vi "MSEncoder Case-22-PhaseScanII.vi"(8 "error in (no error)":errorcluster, 9 "ParamValIn":variant, 11 "MSEncoder in":refnum<class "MSEncoder.lvclass">) -> (0 "error out":errorcluster, 3 "MSEncoder out":refnum<class "MSEncoder.lvclass">)   [LabVIEW 2018, in "MSEncoder.lvclass"]
uses:
  MSEncoder.lvclass
  Ctl/MSEditorParam phaseScanII.ctl
  PublicSubVI/Ctl/MathieuEqParam.ctl
  MSEncoder.lvclass/MSEncoder.ctl
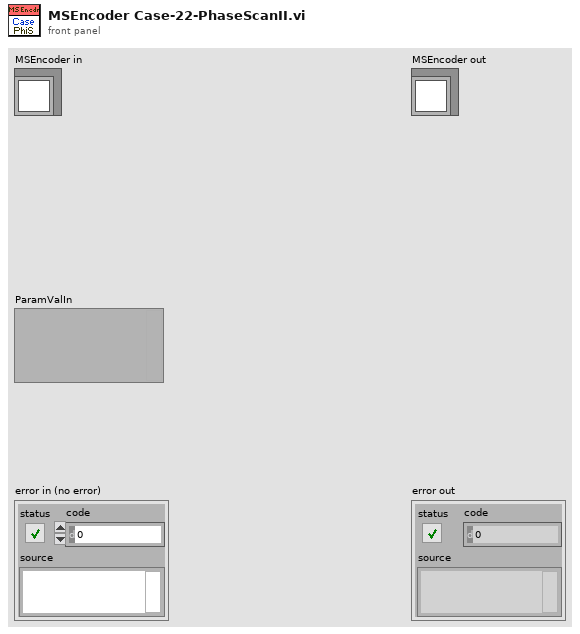
[diagram p1: front panel]
types:
  T1 = typedef "MSEditorParam phaseScanII.ctl" = cluster{"auxWfmType":u32, "auxStart":u32, "iauxCyc":ext, "auxCyc":ext, "beta":ext, "betaScale":ext, "auxAmp":ext, "auxPulse1":ext[], "auxPulse2":ext[], "auxPulseAmp":ext[], "dm":ext, "freq":ext[], "stepWidth":u32}
  T2 = cluster{"f1":ext, "m1":ext, "f2":ext, "Stepwise":u32, "dm":ext}
  T3 = typedef "MathieuEqParam.ctl" = cluster{"mz(Th)":ext, "Amp(V)":ext, "Freq(Hz)":ext, "Beta":ext, "r_0 (mm)":ext, "z_0 (mm)":ext}
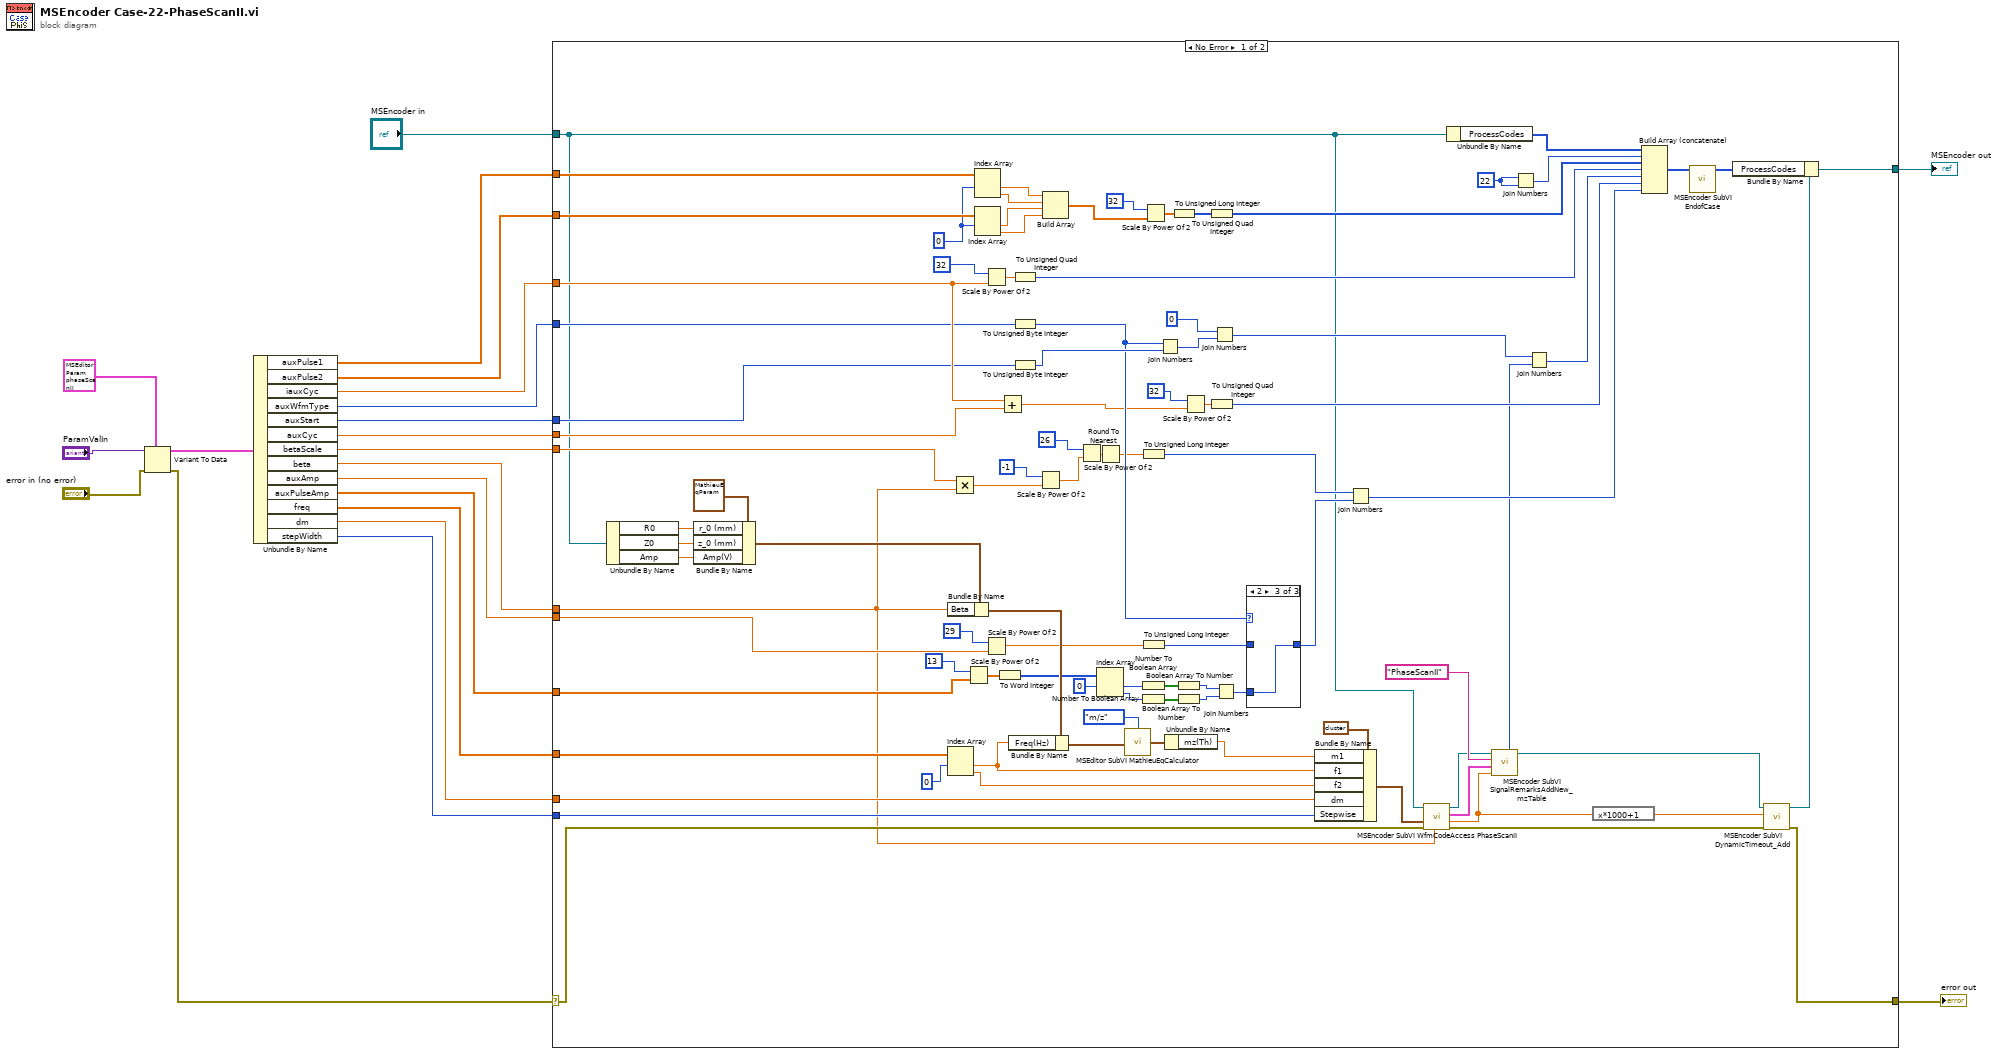
[diagram p0: block diagram]
diagram:
  n1 = Variant To Data(error in="error in (no error)", type=T1 {"auxWfmType"=0, "auxStart"=0, "iauxCyc"=0.0, "auxCyc"=0.0, "beta"=0.5, "betaScale"=1.0, "auxAmp"=1.0, "auxPulse1"=[0.0, 0.5], "auxPulse2"=[0.5, 1.0], "auxPulseAmp"=[1.0, -1.0], "dm"=1.0, "freq"=[100000.0, 50000.0], "stepWidth"=1} ("ParamValueType"), Variant="ParamValIn") -> (data=w3:T1, error out=w2:errorcluster)
  n2 = Unbundle By Name(w3) -> ("auxPulse1"=w20:ext[], "auxPulse2"=w19:ext[], "iauxCyc"=w18:ext, "auxWfmType"=w17:u32, "auxStart"=w16:u32, "auxCyc"=w15:ext, "betaScale"=w14:ext, "beta"=w13:ext, "auxAmp"=w12:ext, "auxPulseAmp"=w11:ext[], "freq"=w10:ext[], "dm"=w9:ext, "stepWidth"=w8:u32)
  n3 = case shown="No Error" w2 {
    selector: w2 -> [w37 w118]
    tunnel: "MSEncoder in" -> [w34 w117]
    tunnel: [w39 w118] -> w21
    tunnel: [w113 w117] -> w6
    tunnel: w20 -> [w107 _]
    tunnel: w19 -> [w106 _]
    tunnel: w18 -> [w105 _]
    tunnel: w17 -> [w104 _]
    tunnel: w16 -> [w103 _]
    tunnel: w15 -> [w102 _]
    tunnel: w14 -> [w101 _]
    tunnel: w13 -> [w22 _]
    tunnel: w12 -> [w100 _]
    tunnel: w11 -> [w99 _]
    tunnel: w10 -> [w98 _]
    tunnel: w9 -> [w26 _]
    tunnel: w8 -> [w25 _]
    frame No Error {
      w90 = u32 22
      w85 = 0 ("index")
      n4 = Unbundle By Name(w34) -> ("R0"=w112:ext, "Z0"=w111:ext, "Amp"=w110:ext)
      n5 = Bundle By Name(cluster=T3 {"mz(Th)"=0.0, "Amp(V)"=330.0, "Freq(Hz)"=0.0, "Beta"=1.0, "r_0 (mm)"=10.0, "z_0 (mm)"=7.0710678118654755} ("Parametres in"), "r_0 (mm)"=w112, "z_0 (mm)"=w111, "Amp(V)"=w110) -> (w108:T3)
      n6 = Bundle By Name(cluster=w108, "Beta"=w22) -> (w97:T3)
      n7 = Index Array(array=w98, index #1=0 ("index")) -> (element #1=w28:ext, element #2=w27:ext)  [unwired: 1 in]
      n8 = Multiply(x=w101, y=w22) -> (x*y=w57:ext)
      n9 = Scale By Power Of 2(n=i16 13, x=w99) -> (x*2^n=w55:ext[])
      n10 = Index Array(array=w107, index #1=w85) -> (element #1=w83:ext, element #2=w82:ext)  [unwired: 1 in]
      n11 = Index Array(array=w106, index #1=w85) -> (element #1=w81:ext, element #2=w80:ext)  [unwired: 1 in]
      n12 = Scale By Power Of 2(n=i16 32, x=w105) -> (x*2^n=w87:ext)
      n13 = Scale By Power Of 2(n=i16 29, x=w100) -> (x*2^n=w60:ext)
      n14 = To Word Integer(number=w55) -> (16bit integer=w54:i16[])
      n15 = Add(x=w105, y=w102) -> (x+y=w43:ext)
      n16 = Bundle By Name(cluster=w97, "Freq(Hz)"=w28) -> (w84:T3)
      n17 = To Unsigned Quad Integer(1:w87) -> (0:w74:u64)
      n18 = To Unsigned Byte Integer(number=w104) -> (unsigned 8bit integer=w47:u8)
      n19 = To Unsigned Byte Integer(number=w103) -> (unsigned 8bit integer=w73:u8)
      n20 = Scale By Power Of 2(n=i16 -1, x=w57) -> (x*2^n=w63:ext)
      n21 = Build Array(w83, w82, w81, w80) -> (w78:ext[])
      n22 = Scale By Power Of 2(n=i16 26, x=w63) -> (x*2^n=w61:ext)
      n23 = Round To Nearest(number=w61) -> (nearest integer value=w42:ext)
      n24 = Index Array(array=w54, index #1=0 ("index")) -> (element #1=w53:i16, element #2=w52:i16)  [unwired: 1 in]
      n25 = call "MSEditor SubVI MathieuEqCalculator.vi"("Target (Freq)"=enum16{"m/z", "Volt", "Freq", "Beta"}."m/z", "Parametres in"=w84) -> ("Parametres out"=w92:T3)  [unwired: 2 in]
      n26 = To Unsigned Long Integer(number=w42) -> (unsigned 32bit integer=w59:u32)
      n27 = To Unsigned Long Integer(number=w60) -> (unsigned 32bit integer=w45:u32)
      n28 = Number To Boolean Array(number=w53) -> (Boolean array=w51:bool[])
      n29 = Number To Boolean Array(number=w52) -> (Boolean array=w50:bool[])
      n30 = Scale By Power Of 2(n=i16 32, x=w78) -> (x*2^n=w77:ext[])
      n31 = Join Numbers(hi=w47, lo=w73) -> ((hi.lo)=w72:u16)
      n32 = Unbundle By Name(w92) -> ("mz(Th)"=w29:ext)
      n33 = To Unsigned Long Integer(number=w77) -> (unsigned 32bit integer=w76:u32[])
      n34 = Boolean Array To Number(Boolean array=w51) -> (number=w48:u16)
      n35 = Boolean Array To Number(Boolean array=w50) -> (number=w49:u16)
      n36 = Scale By Power Of 2(n=i16 32, x=w43) -> (x*2^n=w68:ext)
      n37 = To Unsigned Quad Integer(1:w76) -> (0:w75:u64[])
      n38 = To Unsigned Quad Integer(1:w68) -> (0:w66:u64)
      n39 = Join Numbers(hi=u16 0, lo=w72) -> ((hi.lo)=w70:u32)
      n40 = Join Numbers(hi=w48, lo=w49) -> ((hi.lo)=w46:u32)
      n41 = case shown="2" w47 {
        tunnel: w46 -> [_ _ w116]
        tunnel: w45 -> [w114 w115 _]
        tunnel: [w114 w115 w116] -> w44
        frame 0, Default {
        }
        frame 1 {
        }
        frame 2 {
        }
      }
      n42 = Bundle By Name(cluster=T2 {"f1"=0.0, "m1"=0.0, "f2"=0.0, "Stepwise"=0, "dm"=0.0} ("Data in"), "m1"=w29, "f1"=w28, "f2"=w27, "dm"=w26, "Stepwise"=w25) -> (w30:T2)
      n43 = Join Numbers(hi=w59, lo=w44) -> ((hi.lo)=w58:u64)
      n44 = call "MSEncoder SubVI WfmCodeAccess PhaseScanII.vi"("beta"=w22, "error in"=w37, "Data in"=w30, "MSEncoder in"=w34) -> ("error out"=w38:errorcluster, "Scan time"=w32:dbl, "mzTable"=w35:cluster{"t":dbl[], "mz":dbl[], "beta":dbl[]}, "MSEncoder out"=w24:refnum<class "MSEncoder.lvclass">)  [unwired: 4 in]
      n45 = Unbundle By Name(w34) -> ("ProcessCodes"=w86:u64[])
      n46 = call "MSEncoder SubVI SignalRemarksAddNew_mzTable.vi"("Scan time"=w32, "mzTable"=w35, "Label"="PhaseScanII", "MSEncoder in"=w24) -> ("MSEncoder out"=w23:refnum<class "MSEncoder.lvclass">, "Len"=w36:u32)  [unwired: 6 in]
      n47 = Join Numbers(hi=w90, lo=w90) -> ((hi.lo)=w96:u64)
      n48 = Join Numbers(hi=w70, lo=w36) -> ((hi.lo)=w69:u64)
      n49 = expression code="x*1000+1"(w32) -> (w40:dbl)
      n50 = Build Array (concatenate)(w86, w96, w75, w74, w69, w66, w58) -> (w95:u64[])
      n51 = call "MSEncoder SubVI EndofCase.vi"("Case codes"=w95) -> ("Case codes with end"=w94:u64[])  [unwired: 9 in, 1 out]
      n52 = call "MSEncoder SubVI DynamicTimeout_Add.vi"("error in (no error)"=w38, "Timeout_ms"=w40, "MSEncoder"=w23) -> ("error out"=w39:errorcluster, "MSEncoder"=w41:refnum<class "MSEncoder.lvclass">)  [unwired: 7 in]
      n53 = Bundle By Name(cluster=w41, "ProcessCodes"=w94) -> (w113:refnum<class "MSEncoder.lvclass">)
    }
    frame Error {
    }
  }
  "error out" <- w21
  "MSEncoder out" <- w6
